vi "Z_ROI_compiler-Adjust for short MovCor acquisition cycles26_01_18.vi"(0 "Number of POIs":i32, 1 "Cycle time (us)":dbl, 2 "dISABLE":bool, 5 "Total number of miniscans":i32, 7 "Number of cycles":u64, 9 "ROI Attributes":T1[](array[typedef]) {"Apparent Frame Size" format="%#_6f"; "Original FOV (um)" format="%#_6f"; "Pixels per miniscan" format="%#_6f"; "Dwell Time per pixel" format="%#_6f"; "Resolution" format="%#_6f"; "ROI group ID" format="%#_6f"; "Laser Power (%)" format="%#_6f"; "Zoom" format="%#_6f"; "Frame Size" format="%#_6f"; "Number of lines" format="%#_6f"; "Composite ID" format="%#_6f"; "Angle (deg)" format="%#_6f"; "ROI Time (ns)" format="%#_6f"; "ROI ID" format="%#_6f"; "Pixels in ROI" format="%#_6f"; "ROI index" format="%#_6f"; "Z stop" format="%#_6f"; "Y stop" format="%#_6f"; "X stop" format="%#_6f"; "Z start" format="%#_6f"; "X start" format="%#_6f"; "Y start" format="%#_6f"}, 11 "ROI Attributes (broken down to miniscans) in":T1[](array[typedef]) {"Apparent Frame Size" format="%#_6f"; "Original FOV (um)" format="%#_6f"; "Pixels per miniscan" format="%#_6f"; "Dwell Time per pixel" format="%#_6f"; "Resolution" format="%#_6f"; "ROI group ID" format="%#_6f"; "Laser Power (%)" format="%#_6f"; "Zoom" format="%#_6f"; "Frame Size" format="%#_6f"; "Number of lines" format="%#_6f"; "Composite ID" format="%#_6f"; "Angle (deg)" format="%#_6f"; "ROI Time (ns)" format="%#_6f"; "ROI ID" format="%#_6f"; "Pixels in ROI" format="%#_6f"; "ROI index" format="%#_6f"; "Z stop" format="%#_6f"; "Y stop" format="%#_6f"; "X stop" format="%#_6f"; "Z start" format="%#_6f"; "X start" format="%#_6f"; "Y start" format="%#_6f"}, 12 "ROI Coordinates (broken down to miniscans) in":T2, 13 "Zoom":dbl[](array[numeric])) -> (3 "Cycle time (us) (multiplied by number of stacked cycles)":dbl, 4 "Number of POIs (multiplied by number of stacked cycles)":i32, 6 "Number of miniscans (multiplied by number of stacked cycles)":i32, 8 "Number of cycles or number of stacked cycles":u64, 10 "Zoom":dbl[](array[numeric]), 14 "ROI Coordinates (broken down to miniscans) out":T2, 15 "ROI Attributes (broken down to miniscans) out":T1[](array[typedef]) {"Apparent Frame Size" format="%#_6f"; "Original FOV (um)" format="%#_6f"; "Pixels per miniscan" format="%#_6f"; "Dwell Time per pixel" format="%#_6f"; "Resolution" format="%#_6f"; "ROI group ID" format="%#_6f"; "Laser Power (%)" format="%#_6f"; "Zoom" format="%#_6f"; "Frame Size" format="%#_6f"; "Number of lines" format="%#_6f"; "Composite ID" format="%#_6f"; "Angle (deg)" format="%#_6f"; "ROI Time (ns)" format="%#_6f"; "ROI ID" format="%#_6f"; "Pixels in ROI" format="%#_6f"; "ROI index" format="%#_6f"; "Z stop" format="%#_6f"; "Y stop" format="%#_6f"; "X stop" format="%#_6f"; "Z start" format="%#_6f"; "X start" format="%#_6f"; "Y start" format="%#_6f"})   [LabVIEW 2020]
uses:
  User Interface/Visualisation/Functional Imaging Viewer/Typedefs/ROI parameters data type.ctl
  Typedefs/ROI XY coordinates cluster.ctl
  Typedefs/Imaging Protocols enum.ctl
  Peripherals Control/Pockels/Typedefs/Pockels modulation Internal cluster 1.ctl
  Typedefs/Rounding type.ctl
  Global Variables/General Globals.vi
  Peripherals Control/Pockels/Globals/gl_Pockels control globals.vi
panel:
  in  "Acquisition length (sec)":dbl
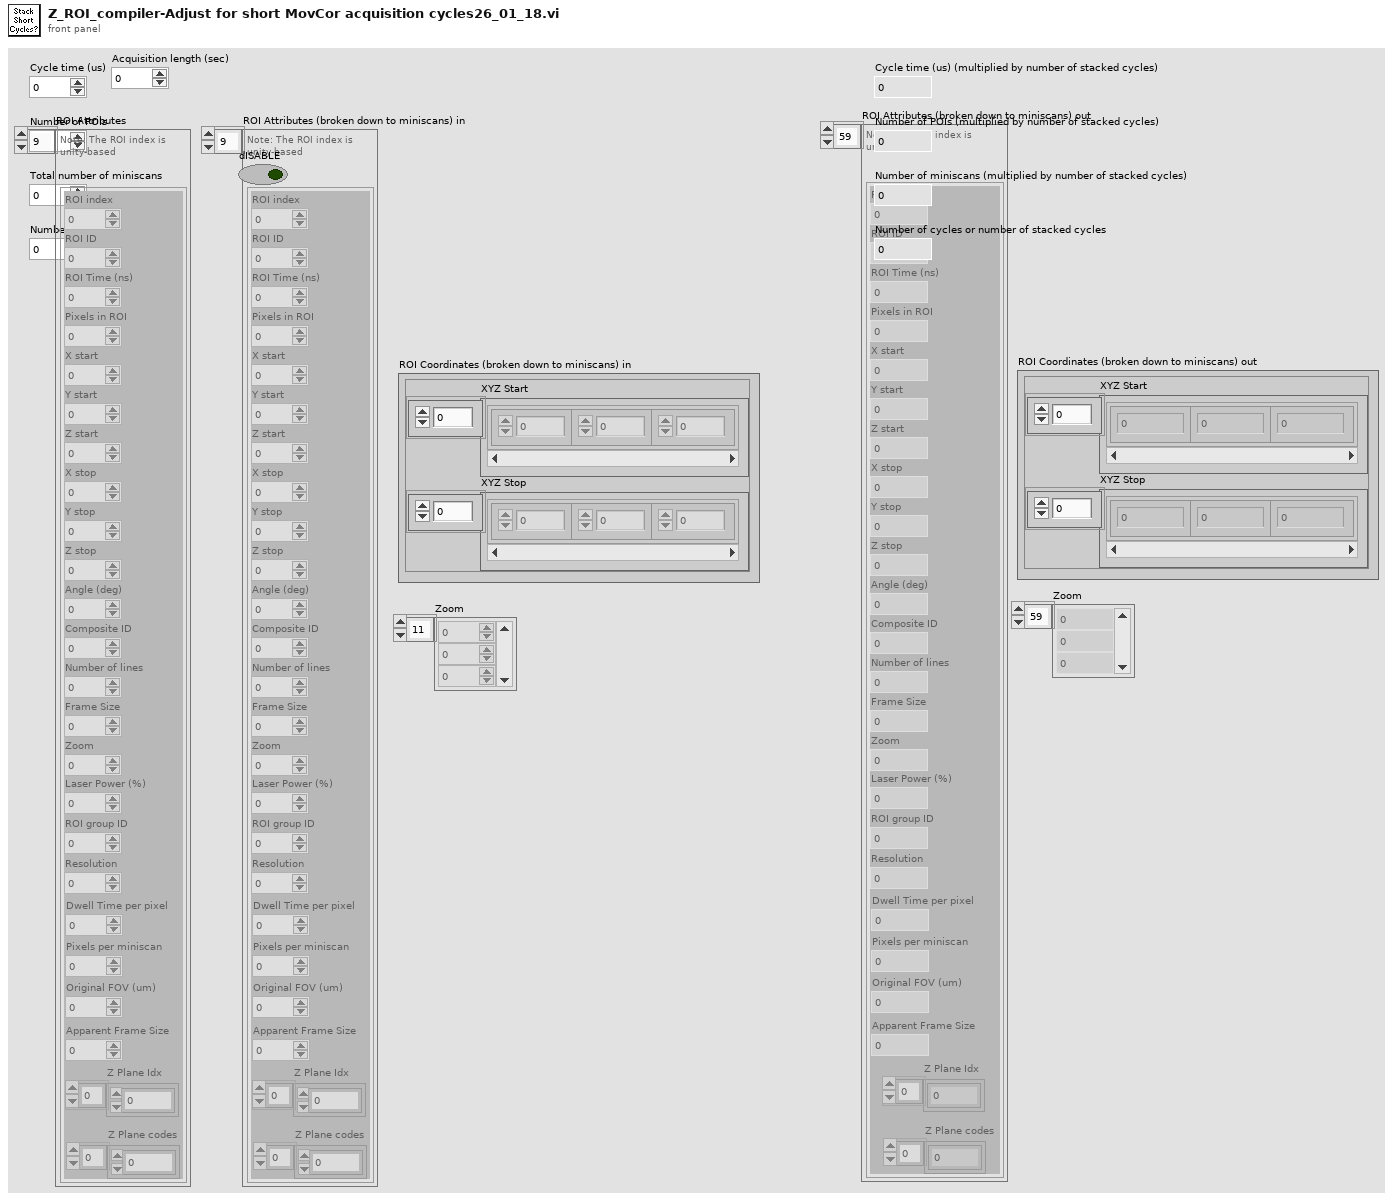
[diagram p1: front panel]
types:
  T1 = typedef "ROI parameters data type.ctl" = cluster{"ROI index":dbl, "ROI ID":dbl, "ROI Time (ns)":dbl, "Pixels in ROI":dbl, "X start":dbl, "Y start":dbl, "Z start":dbl, "X stop":dbl, "Y stop":dbl, "Z stop":dbl, "Angle (deg)":dbl, "Composite ID":dbl, "Number of lines":dbl, "Frame Size":dbl, "Zoom":dbl, "Laser Power (%)":dbl, "ROI group ID":dbl, "Resolution":dbl, "Dwell Time per pixel":dbl, "Pixels per miniscan":dbl, "Original FOV (um)":dbl, "Apparent Frame Size":dbl, "Z Plane Idx":i32[], "Z Plane codes":i32[]}
  T2 = typedef "ROI XY coordinates cluster.ctl" = cluster{"XYZ Start":cluster{"X":sgl, "Y":sgl, "Z":sgl}[], "XYZ Stop":cluster{"X":sgl, "Y":sgl, "Z":sgl}[]}
  T3 = typedef "Pockels modulation Internal cluster 1.ctl" = cluster{"Pockels ON \"Pre\" (samples)":i32, "Direction (+-Inf)":T4, "Additional duration to stay ON (samples)":i32, "Not the last ROI":bool}
  T4 = typedef "Rounding type.ctl" = enum16{"No rounding", "Toward +Inf", "Toward -Inf"}
  T5 = typedef "Imaging Protocols enum.ctl" = enum16{"AOL Z-Stack", "Motor Z Stack", "Functional Acquisition", "Single Plane Acquisition", "Volume Acquisition", "Live Imaging", "Live Plane Imaging", "Live Volume Imaging"}
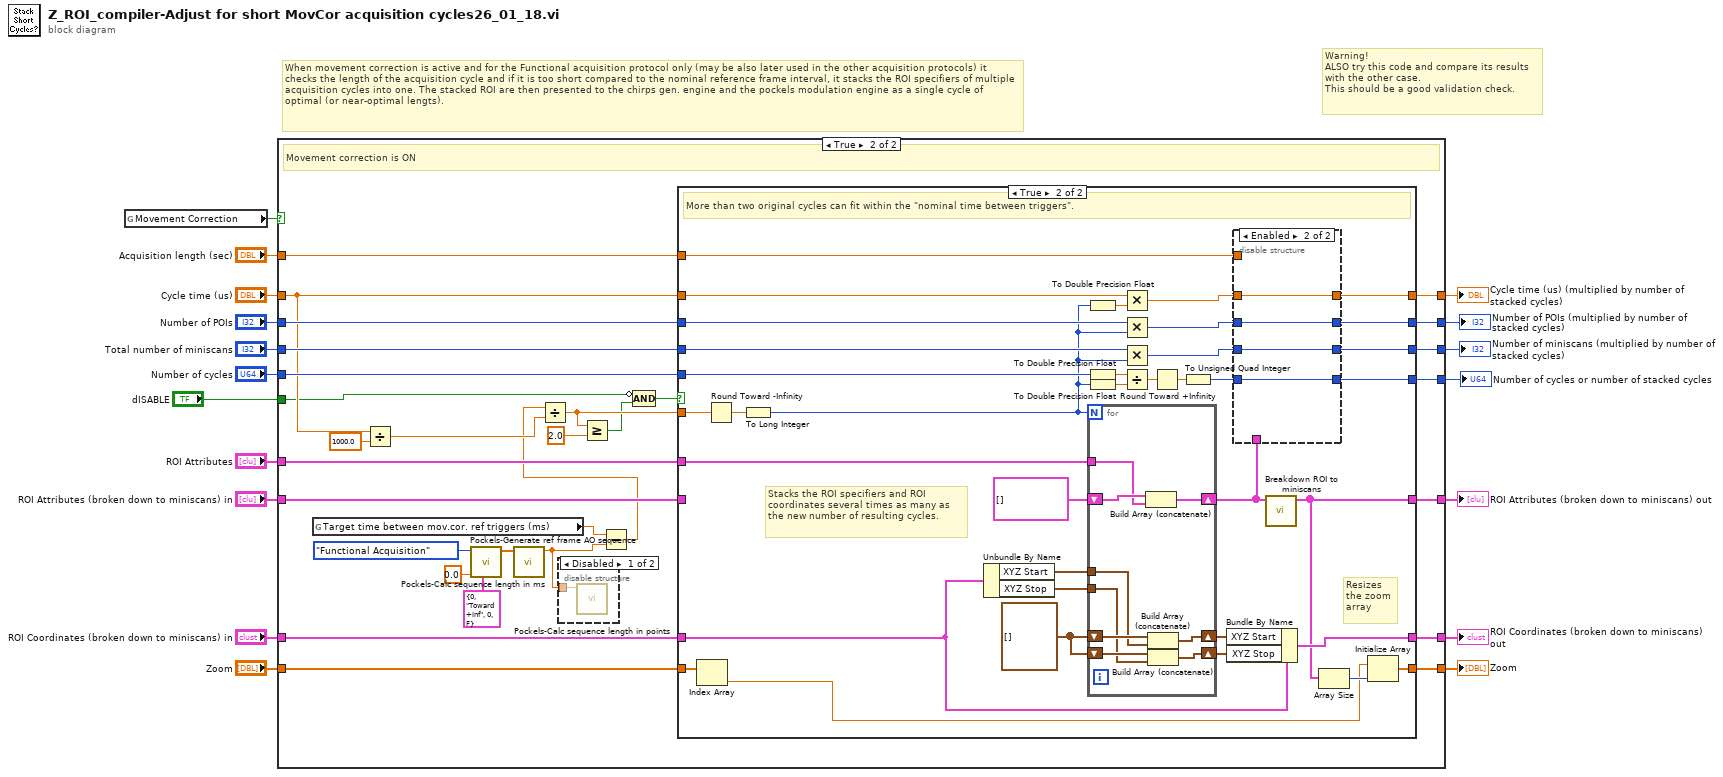
[diagram p0: block diagram]
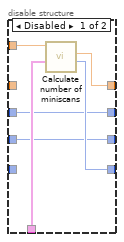
[diagram p5: hidden frame]
diagram:
  # "Warning!\nALSO try this code and compare its results with the other case.\nThis should be a good validation check."
  # "When movement correction is active and for the Functional acquisition protocol only (may be also later used in the other acquisition protocols) it checks the length of the acquisition cycle and if it is too short compared to the nominal reference frame interval, it stacks the ROI specifiers of multiple acquisition cycles into one. The stacked ROI are then presented to the chirps gen. engine and the pockels modulation engine as a single cycle of optimal (or near-optimal lengts)."
  n1 = global read "General Globals.vi" "Movement Correction"() -> (w8:bool)
  n2 = case shown="True" w8 {
    tunnel: "Cycle time (us)" -> [w25 w39]
    tunnel: "ROI Attributes" -> [_ w55]
    tunnel: "Number of cycles" -> [w20 w46]
    tunnel: "ROI Coordinates (broken down to miniscans) in" -> [w23 w54]
    tunnel: [w24 w53] -> w10
    tunnel: [w23 w52] -> w11
    tunnel: [w25 w51] -> w12
    tunnel: "ROI Attributes (broken down to miniscans) in" -> [w24 w43]
    tunnel: [w22 w50] -> w14
    tunnel: "Total number of miniscans" -> [w22 w49]
    tunnel: "Number of POIs" -> [w21 w48]
    tunnel: [w21 w47] -> w17
    tunnel: [w20 w45] -> w18
    tunnel: "Acquisition length (sec)" -> [_ w38]
    tunnel: "Zoom" -> [w19 w36]
    tunnel: [w19 w37] -> w2
    tunnel: "dISABLE" -> [_ w27]
    frame False {
      # "No movement correction"
    }
    frame True {
      # "Movement correction is ON"
      n3 = global read "gl_Pockels control globals.vi" "Target time between mov.cor. ref triggers (ms)"() -> (w34:dbl)
      n4 = Divide(x=w39, y=1000.0) -> (x/y=w40:dbl)
      n5 = call "Pockels-Generate ref frame AO sequence.vi"("Cluster"=T3 {"Pockels ON \"Pre\" (samples)"=0, "Direction (+-Inf)"=enum."Toward +Inf", "Additional duration to stay ON (samples)"=0, "Not the last ROI"=FALSE}, "Previous excess us (us)"=0.0, "Imaging Protocol"=Imaging_Protocols_enum."Functional Acquisition") -> ("Pockels modulation sequence"=w33:dbl[])  [unwired: 4 in, 4 out]
      n6 = call "Pockels-Calc sequence length in ms.vi"("Pockels modulation sequence in"=w33) -> ("Sequence length (ms)"=w35:dbl)  [unwired: 8 in, 2 out]
      n7 = disable-structure shown="Disabled" {
        disable-tunnel: w35 -> [w56 _]
        frame Disabled {
          n8 = call "Pockels-Calc sequence length in points.vi"("Sequence length (ms)"=w56) -> ()  [unwired: 10 in, 1 out]
        }
        frame Enabled {
        }
      }
      n9 = Subtract(x=w34, y=w35) -> (x-y=w29:dbl)
      n10 = Divide(x=w29, y=w40) -> (x/y=w42:dbl)
      n11 = Greater Or Equal?(x=w42, y=2.0) -> (x >= y?=w28:bool)
      n12 = Compound Arithmetic op=AND(invert w27, w28) -> (w26:bool)
      n13 = case shown="True" w26 {
        tunnel: w55 -> [_ w99]
        tunnel: w54 -> [w58 w98]
        tunnel: [w59 w66] -> w53
        tunnel: [w58 w69] -> w52
        tunnel: [w63 w77] -> w51
        tunnel: [w61 w71] -> w50
        tunnel: w49 -> [w61 w97]
        tunnel: w48 -> [w62 w96]
        tunnel: [w62 w70] -> w47
        tunnel: w46 -> [w60 w95]
        tunnel: [w60 w72] -> w45
        tunnel: w39 -> [w63 w94]
        tunnel: w43 -> [w59 _]
        tunnel: w42 -> [_ w93]
        tunnel: w38 -> [_ w78]
        tunnel: [w57 w64] -> w37
        tunnel: w36 -> [w57 w68]
        frame False {
          # "Less than two original cycles fit within the nominal time between triggers."
        }
        frame True {
          w83 = cluster{"X":sgl, "Y":sgl, "Z":sgl}[] [] ("XYZ Coordinates")
          # "Resizes\nthe zoom\narray"
          # "Stacks the ROI specifiers and ROI coordinates several times as many as the new number of resulting cycles."
          # "More than two original cycles can fit within the \"nominal time between triggers\"."
          n14 = Index Array(array=w68) -> (element=w65:dbl)  [unwired: 1 in]
          n15 = Round Toward -Infinity(1:w93) -> (0:w92:dbl)
          n16 = To Long Integer(number=w92) -> (32bit integer=w91:i32)
          n17 = Unbundle By Name(w98) -> ("XYZ Start"=w85:cluster{"X":sgl, "Y":sgl, "Z":sgl}[], "XYZ Stop"=w84:cluster{"X":sgl, "Y":sgl, "Z":sgl}[])
          n18 = To Double Precision Float(number=w91) -> (double precision float=w90:dbl)
          n19 = To Double Precision Float(number=w95) -> (double precision float=w88:dbl)
          n20 = To Double Precision Float(number=w91) -> (double precision float=w87:dbl)
          n21 = for {
            N: w91 -> [_]
            tunnel: w99 -> [w116]
            shift-right: [w117] -> w79
            shift-left: T1[] [] -> [w118]
            tunnel: w85 -> [w111]
            tunnel: w84 -> [w110]
            shift-right: [w113] -> w82
            shift-left: w83 -> [w114]
            shift-right: [w112] -> w81
            shift-left: w83 -> [w115]
            n22 = Build Array (concatenate)(w118, w116) -> (w117:T1[])
            n23 = Build Array (concatenate)(w114, w111) -> (w113:cluster{"X":sgl, "Y":sgl, "Z":sgl}[])
            n24 = Build Array (concatenate)(w115, w110) -> (w112:cluster{"X":sgl, "Y":sgl, "Z":sgl}[])
          }
          n25 = Multiply(x=w94, y=w90) -> (x*y=w76:dbl)
          n26 = Multiply(x=w96, y=w91) -> (x*y=w75:i32)
          n27 = Multiply(x=w97, y=w91) -> (x*y=w74:i32)
          n28 = Divide(x=w88, y=w87) -> (x/y=w89:dbl)
          n29 = Round Toward +Infinity(x=w89) -> (ceil(x): smallest int >= x=w80:dbl)
          n30 = To Unsigned Quad Integer(1:w80) -> (0:w73:u64)
          n31 = Bundle By Name(cluster=w98, "XYZ Start"=w82, "XYZ Stop"=w81) -> (w69:T2)
          n32 = disable-structure shown="Enabled" {
            disable-tunnel: w79 -> [w105 _]
            disable-tunnel: w78 -> [w104 _]
            disable-tunnel: [w103 w109] -> w77
            disable-tunnel: w76 -> [_ w109]
            disable-tunnel: w75 -> [w101 w106]
            disable-tunnel: w74 -> [w100 w107]
            disable-tunnel: w73 -> [_ w108]
            disable-tunnel: [w102 w108] -> w72
            disable-tunnel: [w100 w107] -> w71
            disable-tunnel: [w101 w106] -> w70
            frame Disabled {
              n33 = call "Calculate number of miniscans.vi"("XYZ Coordinates"=w105, "Acquisition length (sec)"=w104) -> ("Number of cycles"=w102:u64, "Cycle time (us)"=w103:dbl)  [unwired: 7 in, 1 out]
            }
            frame Enabled {
            }
          }
          n34 = call "Breakdown ROI to miniscans.vi"("ROI Attributes"=w79) -> ("ROI Attributes (broken down to miniscans)"=w66:T1[])  [unwired: 9 in, 1 out]
          n35 = Array Size(array=w66) -> (size(s)=w67:i32)
          n36 = Initialize Array(w65, w67) -> (w64:dbl[])
        }
      }
    }
  }
  "ROI Attributes (broken down to miniscans) out" <- w10
  "ROI Coordinates (broken down to miniscans) out" <- w11
  "Cycle time (us) (multiplied by number of stacked cycles)" <- w12
  "Number of miniscans (multiplied by number of stacked cycles)" <- w14
  "Number of POIs (multiplied by number of stacked cycles)" <- w17
  "Number of cycles or number of stacked cycles" <- w18
  "Zoom" <- w2
